vi "Source code.vi"() -> ()   [LabVIEW 2021]
uses:
  <vilib>/MakerHub/LINX/Public/Peripherals/Digital/Digital Write 1 Chan.vi
  <vilib>/MakerHub/LINX/Public/Peripherals/PWM/PWM Set Duty Cycle 1 Chan.vi
  <vilib>/MakerHub/LINX/Public/Peripherals/Digital/Digital Write N Chans.vi
  <vilib>/MakerHub/LINX/Private/Local IO/LinxDigitalWrite.vi
  <vilib>/MakerHub/LINX/Public/Utilities/Check Channel.vi
  <vilib>/MakerHub/LINX/Public/Utilities/Open Serial.vi
  <vilib>/MakerHub/LINX/Private/Utilties/Generate Error.vi
  <vilib>/MakerHub/LINX/Public/Peripherals/PWM/PWM Set Duty Cycle N Chans.vi
  <vilib>/MakerHub/LINX/LMH-LINX.lvlib
panel:
  in  "LED SPEED INDICATOR  4":u8
  in  "LED SPEED INDICATOR  2":u8
  in  "LED SPEED INDICATOR  3":u8
  in  "LED SPEED INDICATOR 1":u8
  in  "LED DIRECTION 2":u8
  in  "LED DIRECTION1":u8
  in  "MOTOR DIRECTION":bool
  in  "MOTOR SPEED":dbl(knob) scale=0.0..5.0
  in  "Serial Port":refnum<visa-resource-name>="N/A"
  in  "PWM SPEED":u8
  in  "MOTOR DIRECTION PIN 2":u8
  in  "MOTOR DIRECTION PIN 1":u8
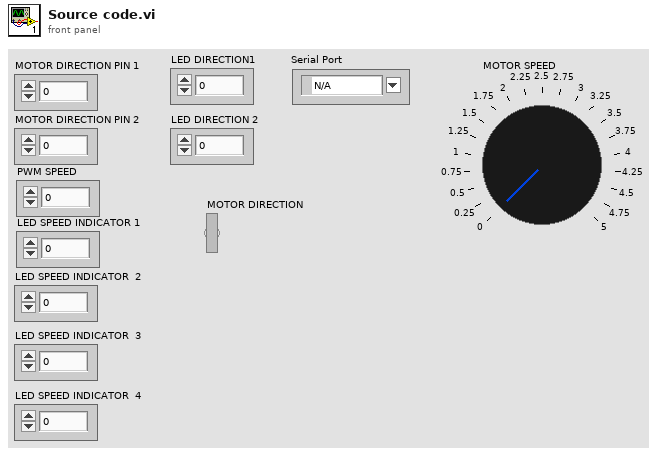
[diagram p1: front panel]
types:
  T1 = typedef "LMH-LINX.lvlib/LINX Ref.ctl" = cluster{"IO":T2, "Interface":T3, "LINX Device Config":T4}
  T2 = typedef "LMH-LINX.lvlib/Platform.ctl" = enum16{"Remote", "Local"}
  T3 = typedef "LMH-LINX.lvlib/Interface.ctl" = enum16{"Serial", "TCP"}
  T4 = typedef "LMH-LINX.lvlib/Device.lvlib/LINX Device Config.ctl" = cluster{"Interface":T3, "COM Port":refnum<visa-resource-name>, "TCP Configuration":T5, "Device Family":u8, "Device ID":u8, "Device Name":string, "TCP Ref":refnum<k5>, "Channels":T6}
  T5 = typedef "LMH-LINX.lvlib/Device.lvlib/TCP Config.ctl" = cluster{"IP Address":string, "Port":u16}
  T6 = typedef "LMH-LINX.lvlib/Channels.ctl" = cluster{"DI":u8[], "DO":u8[], "AI":u8[], "AO":u8[], "PWM":u8[], "QE":u8[], "UART":u8[], "I2C 2":u8[], "SPI":u8[], "CAN":u8[], "Servo":u8[], "AI Ref (V)":dbl, "AI Resolution (Bits)":u8, "AO Ref (V)":dbl, "AO Resolution (Bits)":u8}
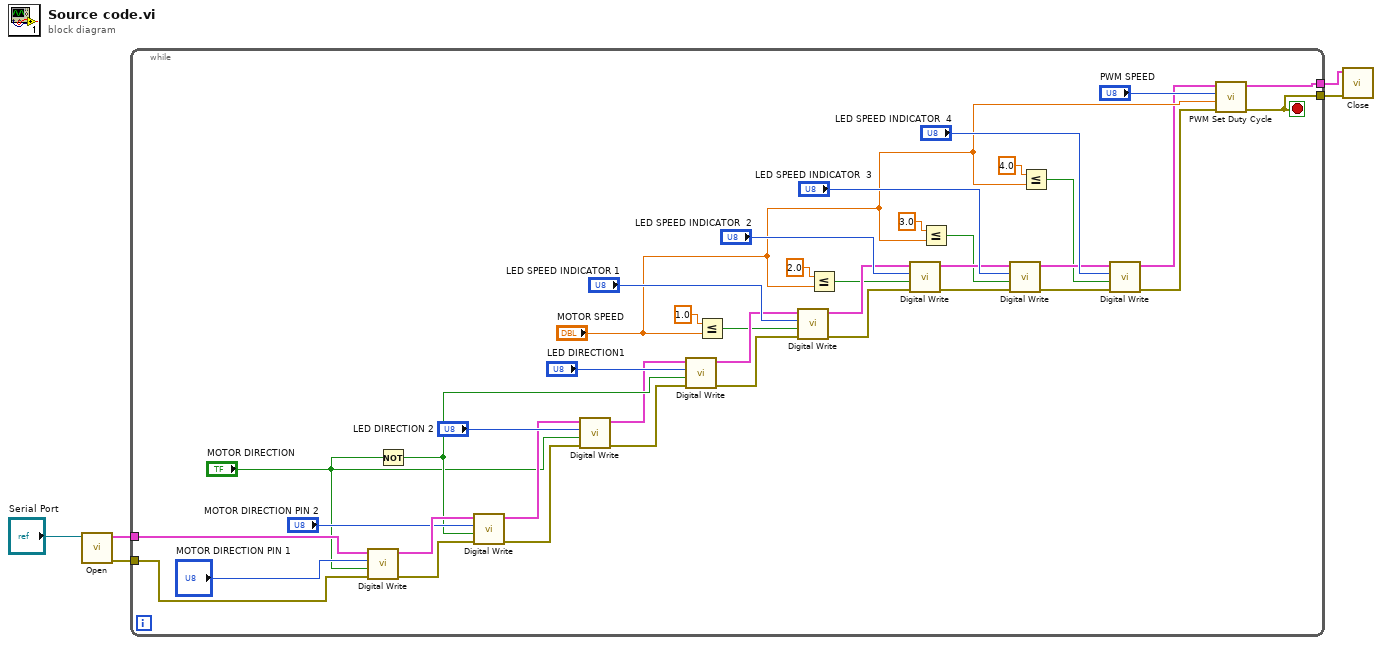
[diagram p0: block diagram]
diagram:
  n1 = call-poly <vilib>:"Open.vi"("Serial Port"="Serial Port") -> ("Error Out"=w3:errorcluster, "LINX Resource"=w5:T1)  [unwired: 8 in, 1 out]
  n2 = while {
    tunnel: w5 -> [w45]
    tunnel: [w39] -> w4
    tunnel: w3 -> [w43]
    tunnel: [w38] -> w2
    stop <- w38 stop-if-true
    n3 = call-poly <vilib>:"Digital Write.vi"("Error In"=w43, "Output Value"="MOTOR DIRECTION", "DO Channel"="MOTOR DIRECTION PIN 1", "LINX Resource"=w45) -> ("Error Out"=w42:errorcluster, "LINX Resource"=w44:T1)  [unwired: 6 in]
    n4 = Not(x="MOTOR DIRECTION") -> (.not. x?=w36:bool)
    n5 = call-poly <vilib>:"Digital Write.vi"("Error In"=w42, "Output Value"=w36, "DO Channel"="MOTOR DIRECTION PIN 2", "LINX Resource"=w44) -> ("Error Out"=w10:errorcluster, "LINX Resource"=w8:T1)  [unwired: 6 in]
    n6 = call-poly <vilib>:"Digital Write.vi"("Error In"=w10, "Output Value"="MOTOR DIRECTION", "DO Channel"="LED DIRECTION 2", "LINX Resource"=w8) -> ("Error Out"=w9:errorcluster, "LINX Resource"=w7:T1)  [unwired: 6 in]
    n7 = call-poly <vilib>:"Digital Write.vi"("Error In"=w9, "Output Value"=w36, "DO Channel"="LED DIRECTION1", "LINX Resource"=w7) -> ("Error Out"=w26:errorcluster, "LINX Resource"=w30:T1)  [unwired: 6 in]
    n8 = Less Or Equal?(x=1.0, y="MOTOR SPEED") -> (x <= y?=w21:bool)
    n9 = call-poly <vilib>:"Digital Write.vi"("Error In"=w26, "Output Value"=w21, "DO Channel"="LED SPEED INDICATOR 1", "LINX Resource"=w30) -> ("Error Out"=w25:errorcluster, "LINX Resource"=w29:T1)  [unwired: 6 in]
    n10 = Less Or Equal?(x=2.0, y="MOTOR SPEED") -> (x <= y?=w17:bool)
    n11 = call-poly <vilib>:"Digital Write.vi"("Error In"=w25, "Output Value"=w17, "DO Channel"="LED SPEED INDICATOR  2", "LINX Resource"=w29) -> ("Error Out"=w24:errorcluster, "LINX Resource"=w28:T1)  [unwired: 6 in]
    n12 = Less Or Equal?(x=3.0, y="MOTOR SPEED") -> (x <= y?=w20:bool)
    n13 = call-poly <vilib>:"Digital Write.vi"("Error In"=w24, "Output Value"=w20, "DO Channel"="LED SPEED INDICATOR  3", "LINX Resource"=w28) -> ("Error Out"=w23:errorcluster, "LINX Resource"=w27:T1)  [unwired: 6 in]
    n14 = Less Or Equal?(x=4.0, y="MOTOR SPEED") -> (x <= y?=w14:bool)
    n15 = call-poly <vilib>:"Digital Write.vi"("Error In"=w23, "Output Value"=w14, "DO Channel"="LED SPEED INDICATOR  4", "LINX Resource"=w27) -> ("Error Out"=w12:errorcluster, "LINX Resource"=w13:T1)  [unwired: 6 in]
    n16 = call-poly <vilib>:"PWM Set Duty Cycle.vi"("Error In"=w12, "Duty Cycle (0-1)"="MOTOR SPEED", "PWM Channel"="PWM SPEED", "LINX Resource"=w13) -> ("Error Out"=w38:errorcluster, "LINX Resource"=w39:T1)  [unwired: 6 in]
  }
  n17 = call <vilib>:"Close.vi"("Error In"=w2, "LINX Resource"=w4) -> ()  [unwired: 9 in, 1 out]
